vi "CAPTH-Init Analysis.vi"(0 "Datafile":path, 5 "Params":T4={"Stimulus"={"EAR"=enum."RIGHT", "HI FREQ"=18.0, "LO FREQ"=5.0, "FREQ STEP"=8, "Rep Rate (/s)"=20.0, "Alternate Polarity"=TRUE, "# CYCLES"=1, "Duration (ms)"=0.0, "Ramp (ms)"=0.0}, "Response"={"Averages (3dB steps)"=12, "Time Window (ms)"=8.5, "dt (us)"=10.0, "Grass gain"=1000.0, "CRITERION (mV)"=60.0, "CEILING (dB atten)"=6.0, "Use previous"=FALSE, "Save avgs"=FALSE, "Save raw"=FALSE, "Save history"=FALSE, "CEILING (dB SPL)"=6.0}} {"Response"."CRITERION (mV)" format="%.2f"; "Response"."Time Window (ms)" format="%.2f"}) -> (4 "State":T1, 15 "error out":errorcluster)   [LabVIEW 2020]
uses:
  Typedefs/CAPTH-Parameters.ctl
  Typedefs/CAPTH-Stimulus.ctl
  Typedefs/CAPTH-Response.ctl
  Typedefs/CAPTH-Analysis State.ctl
  Typedefs/CAPTH-History.ctl
  Typedefs/CAPTH-StimCon.ctl
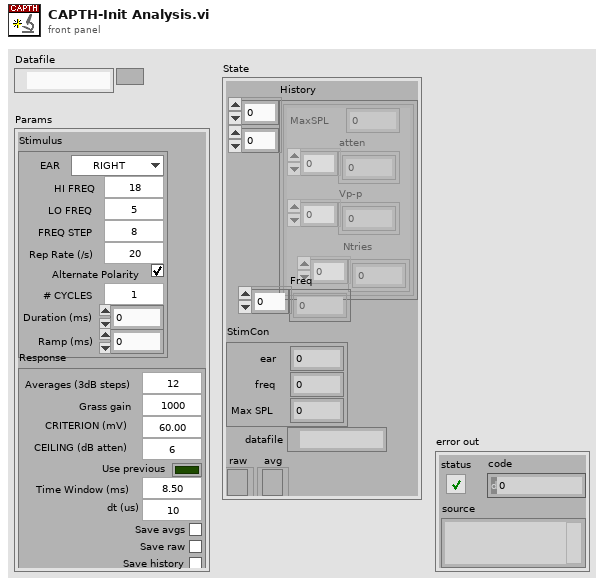
[diagram p1: front panel]
types:
  T1 = typedef "CAPTH-Analysis State.ctl" = cluster{"History":T2, "Freq":dbl[], "StimCon":T3, "datafile":path, "raw":refnum<file>, "avg":refnum<file>}
  T2 = typedef "CAPTH-History.ctl" = cluster{"MaxSPL":dbl, "atten":dbl[], "Vp-p":dbl[], "Ntries":i32[]}[][]
  T3 = typedef "CAPTH-StimCon.ctl" = cluster{"ear":i32, "freq":i32, "Max SPL":dbl}
  T4 = typedef "CAPTH-Parameters.ctl" = cluster{"Stimulus":T5, "Response":T6}
  T5 = typedef "CAPTH-Stimulus.ctl" = cluster{"EAR":enum16{"RIGHT", "LEFT\n", "ALTERNATE"}, "HI FREQ":dbl, "LO FREQ":dbl, "FREQ STEP":u8, "Rep Rate (/s)":dbl, "Alternate Polarity":bool, "# CYCLES":u8, "Duration (ms)":dbl, "Ramp (ms)":dbl}
  T6 = typedef "CAPTH-Response.ctl" = cluster{"Averages (3dB steps)":i32, "Time Window (ms)":dbl, "dt (us)":dbl, "Grass gain":dbl, "CRITERION (mV)":dbl, "CEILING (dB atten)":dbl, "Use previous":bool, "Save avgs":bool, "Save raw":bool, "Save history":bool, "CEILING (dB SPL)":dbl}
  T7 = enum16{"open", "replace", "create", "open or create", "replace or create", "replace or create with confirmation"}
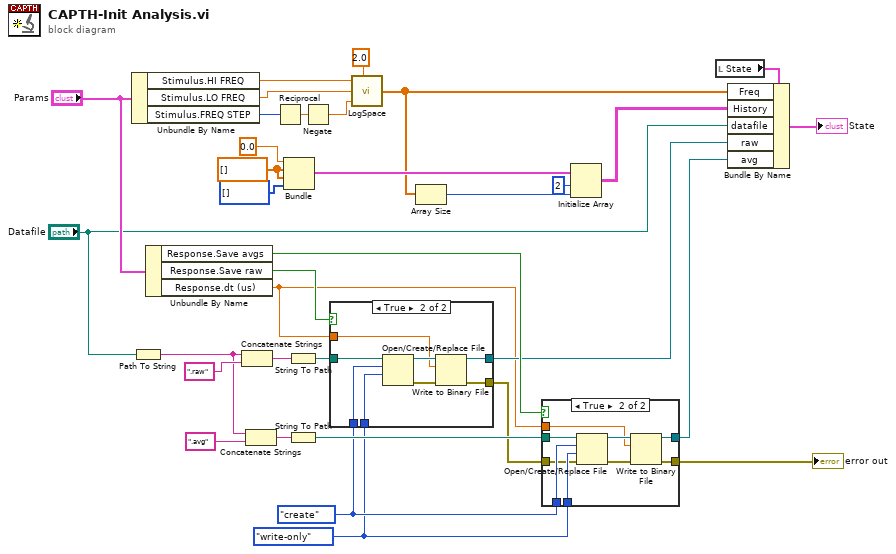
[diagram p0: block diagram]
diagram:
  w8 = enum16{"read/write", "read-only", "write-only"}."write-only" ("access (0:read/write)")
  w9 = T7."create" ("operation (0:open)")
  w27 = dbl[] []
  n1 = Unbundle By Name("Params") -> ("Stimulus.HI FREQ"=w31:dbl, "Stimulus.LO FREQ"=w30:dbl, "Stimulus.FREQ STEP"=w29:u8)
  n2 = Path To String(path="Datafile") -> (string=w18:string)
  n3 = Unbundle By Name("Params") -> ("Response.Save avgs"=w12:bool, "Response.Save raw"=w13:bool, "Response.dt (us)"=w4:dbl)
  n4 = Concatenate Strings(w18, ".raw") -> (w17:string)
  n5 = Concatenate Strings(w18, ".avg" ("string")) -> (w16:string)
  n6 = Reciprocal(x=w29) -> (1/x=w33:dbl)
  n7 = Bundle(0.0, w27, w27, i32[] []) -> (w26:cluster{dbl, dbl[], dbl[], i32[]})  [unwired: 1 in]
  n8 = String To Path(string=w17) -> (path=w14:path)
  n9 = String To Path(string=w16) -> (path=w11:path)
  n10 = Negate(x=w33) -> (-x=w32:dbl)
  n11 = case shown="True" w13 {
    tunnel: w14 -> [_ w42]
    tunnel: [_ w37] -> w6
    tunnel: w9 -> [_ w41]
    tunnel: w8 -> [_ w40]
    tunnel: [_ w36] -> w10
    tunnel: w4 -> [_ w35]
    frame False {
    }
    frame True {
      n12 = Open/Create/Replace File(file path (use dialog)=w42, operation (0:open)=w41, access (0:read/write)=w40) -> (refnum out=w38:refnum<file>, error out=w39:errorcluster)  [unwired: 3 in, 1 out]
      n13 = Write to Binary File(file (use dialog)=w38, data=w35, error in=w39) -> (refnum out=w37:refnum<file>, error out=w36:errorcluster)  [unwired: 3 in, 1 out]
    }
  }
  n14 = call "LogSpace.vi"("Start"=w31, "Base"=2.0, "Stop"=w30, "Step"=w32) -> ("Array"=w24:dbl[])  [unwired: 2 in, 1 out]
  n15 = Array Size(array=w24) -> (size(s)=w25:i32)
  n16 = case shown="True" w12 {
    tunnel: w11 -> [_ w51]
    tunnel: [_ w45] -> w5
    tunnel: w9 -> [_ w50]
    tunnel: w8 -> [_ w49]
    tunnel: [_ w44] -> w7
    tunnel: w10 -> [_ w48]
    tunnel: w4 -> [_ w43]
    frame False {
    }
    frame True {
      n17 = Open/Create/Replace File(file path (use dialog)=w51, error in=w48, operation (0:open)=w50, access (0:read/write)=w49) -> (refnum out=w46:refnum<file>, error out=w47:errorcluster)  [unwired: 2 in, 1 out]
      n18 = Write to Binary File(file (use dialog)=w46, data=w43, error in=w47) -> (refnum out=w45:refnum<file>, error out=w44:errorcluster)  [unwired: 3 in, 1 out]
    }
  }
  "error out" <- w7
  n19 = Initialize Array(w26, 2 ("dimension size"), w25) -> (w22:cluster{dbl, dbl[], dbl[], i32[]}[][])
  n20 = local read "State"() -> (w34:T1)
  n21 = Bundle By Name(cluster=w34, "Freq"=w24, "History"=w22, "datafile"="Datafile", "raw"=w6, "avg"=w5) -> (→"State":T1)
